vi "Initialize update array.vi"(10 "Camera label names":string[](array[string])=["Cam1", "Cam2", "Cam3", "Cam4", "Cam5"], 11 "RBCIA (Rack based camera image indicator mapping) out":cluster{"Rack Id":u8, "Label names":string[]}[](array[cluster])=[{"Rack Id"=0, "Label names"=["Cam1", "Cam2", "Cam3"]}, {"Rack Id"=1, "Label names"=["Cam4", "Cam5"]}]) -> (3 "Dynamic image update params.Image update":cluster{"Rack Id":i32, "Update image":bool[]}[](array[cluster]))   [LabVIEW 2019, in "ZenGage v3.0 UI.lvclass"]
uses:
  ZenGage v3.0 UI.lvclass
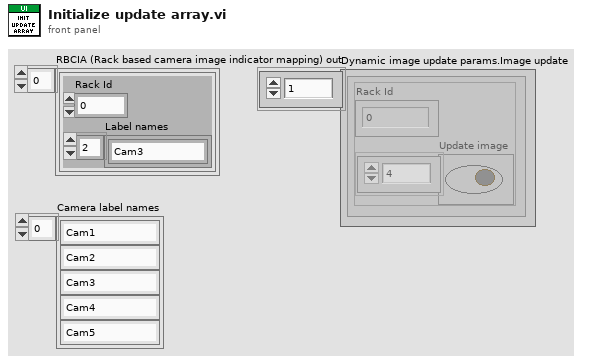
[diagram p1: front panel]
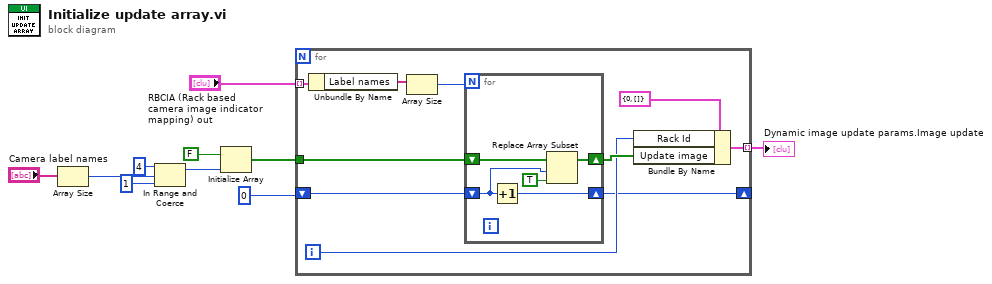
[diagram p0: block diagram]
diagram:
  n1 = Array Size(array="Camera label names") -> (size(s)=w7:i32)
  n2 = In Range and Coerce(upper limit=4, x=w7, lower limit=1) -> (coerced(x)=w4:i32)  [unwired: 1 out]
  n3 = Initialize Array(FALSE, w4) -> (w2:bool[])
  n4 = for {
    tunnel: "RBCIA (Rack based camera image indicator mapping) out" -> [w20] mode=indexing
    tunnel: [w15] -> w3 mode=indexing
    tunnel: w2 -> [w13]
    shift-right: [w11] -> _
    shift-left: 0 -> [w12]
    i -> [w14]
    n5 = Unbundle By Name(w20) -> ("Label names"=w19:string[])
    n6 = Array Size(array=w19) -> (size(s)=w18:i32)
    n7 = for {
      N: w18 -> [_]
      shift-right: [w23] -> w16
      shift-left: w13 -> [w25]
      shift-right: [w22] -> w11
      shift-left: w12 -> [w21]
      n8 = Increment(x=w21) -> (x+1=w22:i32)
      n9 = Replace Array Subset(array=w25, new element=TRUE ("new element/subarray"), index=w21) -> (w23:bool[])
    }
    n10 = Bundle By Name(cluster=cluster{"Rack Id":i32, "Update image":bool[]} {"Rack Id"=0, "Update image"=[]} ("Cluster"), "Rack Id"=w14, "Update image"=w16) -> (w15:cluster{"Rack Id":i32, "Update image":bool[]})
  }
  "Dynamic image update params.Image update" <- w3
